vi "Conversion tension température.vi"(11 "Data In":dbl[](array[numeric])) -> (3 "Data Out":dbl[](array[numeric]))   [LabVIEW 2018]
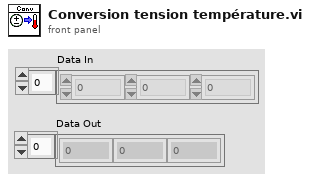
[diagram p1: front panel]
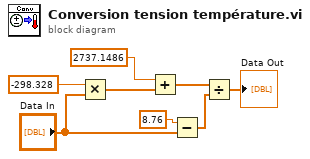
[diagram p0: block diagram]
diagram:
  n1 = Multiply(x=-298.328, y="Data In") -> (x*y=w2:dbl[])
  n2 = Add(x=2737.1486, y=w2) -> (x+y=w1:dbl[])
  n3 = Subtract(x=8.76, y="Data In") -> (x-y=w6:dbl[])
  n4 = Divide(x=w1, y=w6) -> (x/y=→"Data Out":dbl[])
